vi "Units_to_SI_units_converter.vi"(10 "var_value in":dbl, 11 "String in":string) -> (2 "var_value out":dbl, 3 "String out":string)   [LabVIEW 2020]
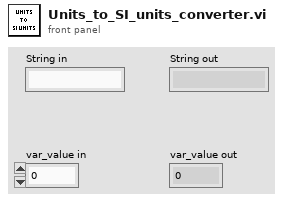
[diagram p1: front panel]
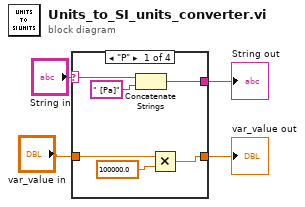
[diagram p0: block diagram]
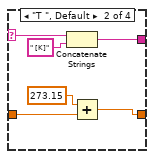
[diagram p2: hidden frame]
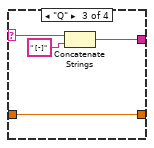
[diagram p3: hidden frame]
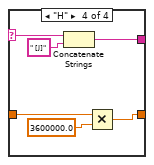
[diagram p4: hidden frame]
diagram:
  n1 = case shown="\"P\"" "String in" {
    selector: "String in" -> [w7 w12 w19 w23]
    tunnel: [w10 w15 w20 w22] -> w1
    tunnel: "var_value in" -> [w8 w14 w20 w24]
    tunnel: [w5 w11 w17 w21] -> w3
    frame "P" {
      n2 = Concatenate Strings(w7, " [Pa]") -> (w5:string)
      n3 = Multiply(x=w8, y=100000.0) -> (x*y=w10:dbl)
    }
    frame "T ", Default {
      n4 = Concatenate Strings(w12, " [K]") -> (w11:string)
      n5 = Add(x=273.15, y=w14) -> (x+y=w15:dbl)
    }
    frame "Q" {
      n6 = Concatenate Strings(w19, " [-]") -> (w17:string)
    }
    frame "H" {
      n7 = Concatenate Strings(w23, " [J]") -> (w21:string)
      n8 = Multiply(x=w24, y=3600000.0) -> (x*y=w22:dbl)
    }
  }
  "String out" <- w3
  "var_value out" <- w1
